vi "一维转化为二维数组.vi"(1 "一维数组":dbl[](array[numeric])) -> (0 "二维数组":dbl[][](array[numeric]))   [LabVIEW 2009]
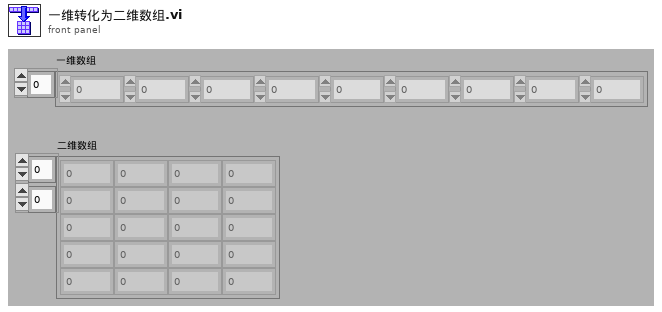
[diagram p1: front panel]
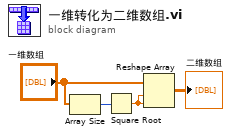
[diagram p0: block diagram]
diagram:
  n1 = Array Size(array="一维数组") -> (size(s)=w3:i32)
  n2 = Square Root(x=w3) -> (sqrt(x)=w1:dbl)
  n3 = Reshape Array("一维数组", w1, w1) -> (→"二维数组":dbl[][])
